vi "Read pathname.vi"(8 "error in (no error)":errorcluster, 11 "Unix Pipe in":refnum<class "Unix Pipe.lvclass">) -> (0 "error out":errorcluster, 2 "pathname":string, 3 "Unix Pipe out":refnum<class "Unix Pipe.lvclass">)   [LabVIEW 2013, in "Pipes.lvlib" / "Unix Pipe.lvclass"]
uses:
  Unix Pipe.lvclass
  Unix Pipe.lvclass/Unix Pipe.ctl
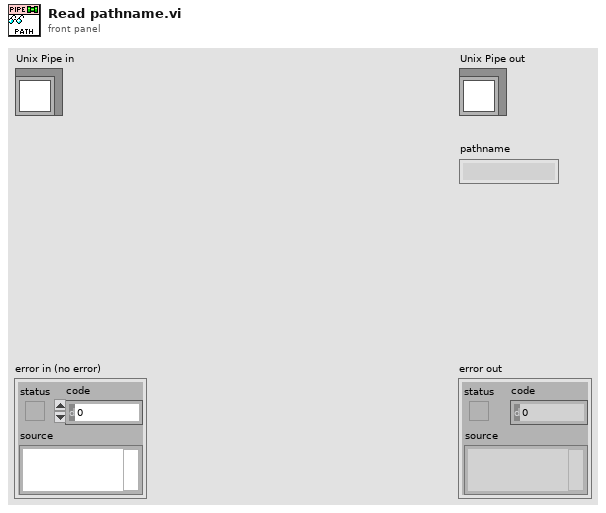
[diagram p1: front panel]
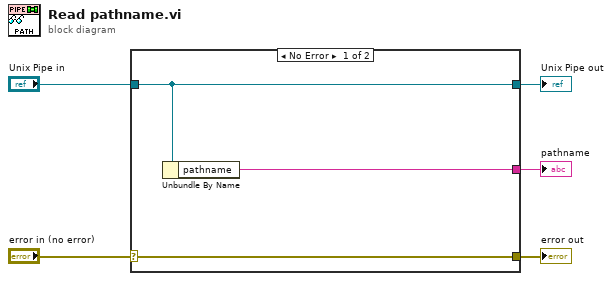
[diagram p0: block diagram]
diagram:
  n1 = case shown="No Error" "error in (no error)" {
    selector: "error in (no error)" -> [w8 w9]
    tunnel: [w8 w9] -> w4
    tunnel: [w7 w10] -> w2
    tunnel: "Unix Pipe in" -> [w7 w10]
    tunnel: [w6 _] -> w1
    frame No Error {
      n2 = Unbundle By Name(w7) -> ("pathname"=w6:string)
    }
    frame Error {
    }
  }
  "error out" <- w4
  "Unix Pipe out" <- w2
  "pathname" <- w1
